vi "Do.vi"(8 "error in":errorcluster, 10 "Actor in":refnum<class "Actor.lvclass">, 11 "Pack Message for Shipping":refnum<class "Pack Message for Shipping .lvclass">) -> (0 "error out":errorcluster, 2 "Actor out":refnum<class "Actor.lvclass">)   [LabVIEW 2014, in "Controller.lvlib" / "Pack Message for Shipping .lvclass"]
doc: "(<B>Filename</B>: Actor Framework.lvlib:Message.lvclass:Do.vi)\n\nDefines what a message does when it is received by an actor. Generally, a message instructs an actor to invoke one of its methods. By default, this method does nothing. A child class must override it to define behavior. Create a child class by using the Actor Framework Message Maker dialog box."
uses:
  Pack Message for Shipping .lvclass
  <vilib>/ActorFramework/Actor/Actor.lvclass
  Controller.lvclass
  <vilib>/ActorFramework/Message Enqueuer/Message Enqueuer.lvclass
  Controls/eMap.ctl
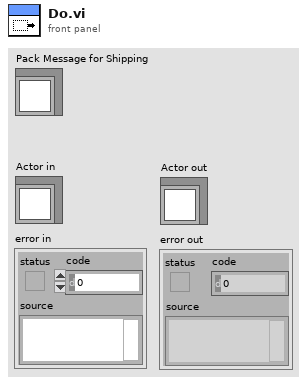
[diagram p1: front panel]
types:
  T1 = typedef "Controller.lvlib/Controller.lvclass/eMap.ctl" = cluster{"Enqueuer":refnum<class "Message Enqueuer.lvclass">, "Active":bool}
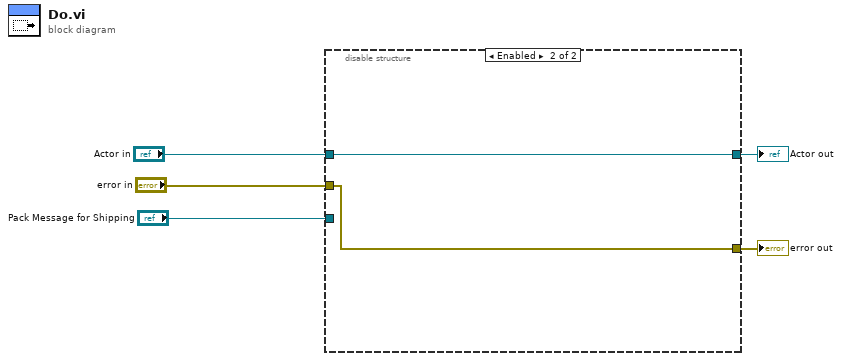
[diagram p0: block diagram]
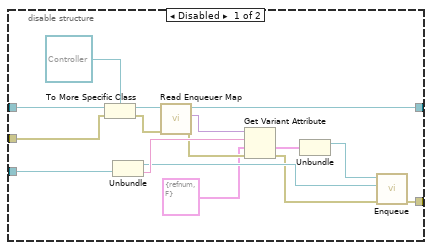
[diagram p2: hidden frame]
diagram:
  n1 = disable-structure shown="Enabled" {
    disable-tunnel: "Actor in" -> [w21 w23]
    disable-tunnel: [w20 w23] -> w4
    disable-tunnel: [w19 w22] -> w3
    disable-tunnel: "error in" -> [w18 w22]
    disable-tunnel: "Pack Message for Shipping" -> [w14 _]
    frame Disabled {
      n2 = To More Specific Class(target class=refnum<class "Controller.lvclass"> refnum ("Controller:Controller"), reference=w21, error in=w18) -> (specific class reference=w16:refnum<class "Controller.lvclass">, error out=w9:errorcluster)
      n3 = Unbundle(w14) -> (w11:refnum<class "Message.lvclass">, w13:string)
      n4 = call "Read Enqueuer Map.vi"("error in (no error)"=w9, "Controller in"=w16) -> ("error out"=w8:errorcluster, "Enqueuer Map"=w15:variant, "Controller out"=w20:refnum<class "Controller.lvclass">)  [unwired: 7 in]
      n5 = Get Variant Attribute(Variant=w15, name=w13, default value (empty Variant)=T1 {"Enqueuer"=refnum, "Active"=FALSE} ("eMap"), error in=w8) -> (value=w12:T1, error out=w7:errorcluster)  [unwired: 2 out]
      n6 = Unbundle(w12) -> ("Enqueuer"=w10:refnum<class "Message Enqueuer.lvclass">)  [unwired: 1 out]
      n7 = call <vilib>:"Enqueue.vi"("error in (no error)"=w7, "Message"=w11, "Message Enqueuer in"=w10) -> ("error out"=w19:errorcluster)  [unwired: 7 in, 1 out]
    }
    frame Enabled {
    }
  }
  "error out" <- w3
  "Actor out" <- w4
